vi "find time.vi"() -> (0 "day":string, 1 "month":string, 2 "year":string)   [LabVIEW 2013]
panel:
  out "日期/时间字符串":string
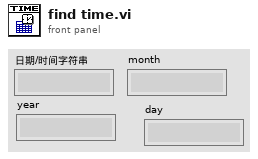
[diagram p1: front panel]
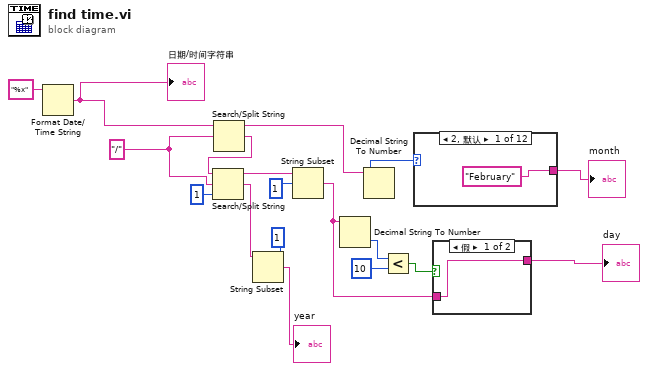
[diagram p0: block diagram]
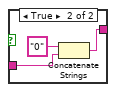
[diagram p2: hidden frame]
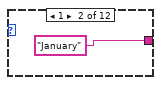
[diagram p3: hidden frame]
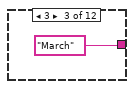
[diagram p4: hidden frame]
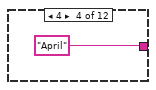
[diagram p5: hidden frame]
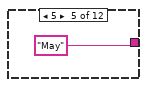
[diagram p6: hidden frame]
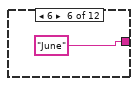
[diagram p7: hidden frame]
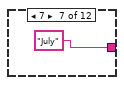
[diagram p8: hidden frame]
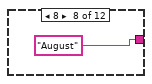
[diagram p9: hidden frame]
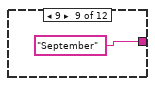
[diagram p10: hidden frame]
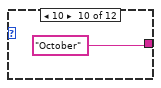
[diagram p11: hidden frame]
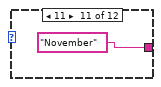
[diagram p12: hidden frame]
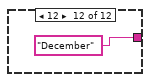
[diagram p13: hidden frame]
diagram:
  w13 = "/" ("搜索字符串/字符(-)")
  n1 = Format Date/Time String(time format string (%c)="%x" ("时间格式字符串(%c)")) -> (date/time string=w17:string)  [unwired: 2 in]
  "日期/时间字符串" <- w17
  n2 = Search/Split String(string=w17, search string/char (-)=w13) -> (substring before match=w3:string, match + rest of string=w16:string)  [unwired: 1 in, 1 out]
  n3 = Search/Split String(string=w16, search string/char (-)=w13, offset (0)=1 ("偏移量(0)")) -> (substring before match=w15:string, match + rest of string=w10:string)  [unwired: 1 out]
  n4 = String Subset(string=w10, offset (0)=1 ("偏移量(0)")) -> (substring=→"year":string)  [unwired: 1 in]
  n5 = String Subset(string=w15, offset (0)=1 ("偏移量(0)")) -> (substring=w2:string)  [unwired: 1 in]
  n6 = Decimal String To Number(string=w2) -> (number=w7:i32)  [unwired: 2 in, 1 out]
  n7 = Decimal String To Number(string=w3) -> (number=w9:i32)  [unwired: 2 in, 1 out]
  n8 = Less?(x=w7, y=10) -> (x < y?=w5:bool)
  n9 = case shown="2, 默认" w9 {
    tunnel: ["February" ("搜索字符串/字符(-)") "January" ("搜索字符串/字符(-)") "March" ("搜索字符串/字符(-)") "April" ("搜索字符串/字符(-)") "May" ("搜索字符串/字符(-)") "June" ("搜索字符串/字符(-)") "July" ("搜索字符串/字符(-)") "August" ("搜索字符串/字符(-)") "September" ("搜索字符串/字符(-)") "October" ("搜索字符串/字符(-)") "November" ("搜索字符串/字符(-)") "December" ("搜索字符串/字符(-)")] -> w8
    frame 2, Default {
    }
    frame 1 {
    }
    frame 3 {
    }
    frame 4 {
    }
    frame 5 {
    }
    frame 6 {
    }
    frame 7 {
    }
    frame 8 {
    }
    frame 9 {
    }
    frame 10 {
    }
    frame 11 {
    }
    frame 12 {
    }
  }
  "month" <- w8
  n10 = case shown="假" w5 {
    tunnel: w2 -> [w31 w33]
    tunnel: [w31 w32] -> w4
    frame False {
    }
    frame True {
      n11 = Concatenate Strings("0" ("搜索字符串/字符(-)"), w33) -> (w32:string)
    }
  }
  "day" <- w4
